vi "trafficlight_Test.vi"() -> ()   [LabVIEW 2022 SP3]
panel:
  in  "stop":bool
  in  "Boolean 3":bool
  in  "Boolean 2":bool
  in  "Boolean":bool
  out "TrafficLight":cluster{"red":bool, "orange":bool, "green":bool}
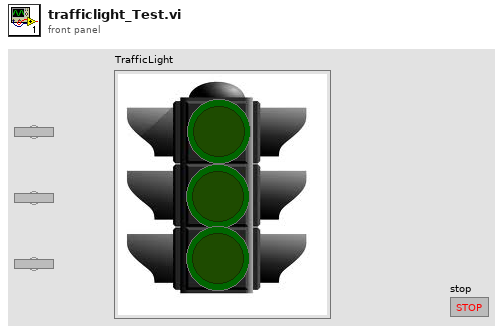
[diagram p1: front panel]
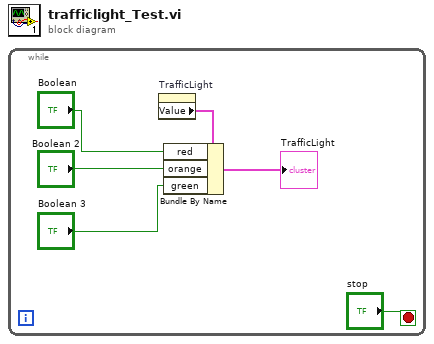
[diagram p0: block diagram]
diagram:
  n1 = while {
    stop <- "stop" stop-if-true
    n2 = property on="TrafficLight" class="Clust (strict)"() -> ("Value"=w6:cluster{"red":bool, "orange":bool, "green":bool})  [unwired: 2 in, 2 out]
    n3 = Bundle By Name(cluster=w6, "red"="Boolean", "orange"="Boolean 2", "green"="Boolean 3") -> (→"TrafficLight":cluster{"red":bool, "orange":bool, "green":bool})
  }
